vi "get_averaging_params_fd.vi"(7 "Current/sensor index":i32 min=0 max=1 step=1, 10 "Modulation info":T3 {"Hi channels at low" min=0 step=1; "Low carriers" format="%#_6p"; "High carriers" format="%#_6p"}, 11 "Config":T4={"IO params"={"Conversion"={"Rate"=4.0, "Num cards"=2, "Out channels"=4}, "Carriers"={"Phase shift"=180.0, "Levels"=[[0.8, 0.8, 0.8], [0.03, 0.03, 0.03]], "Delay samples"=73.15}, "TCP"={"Host"="192.168.1.15", "Port"=6666, "Buffering"=6, "Timeout"=6}, "Input channel sign"=[1, 1, 1]}, "High rate STFT"={"Win param"=101.5, "Window type"=61, "Win order"=2, "DFT size"=64, "Channels"=[7], "Oversample"=64}, "Low rate STFT"={"Win param"=120.0, "Window type"=61, "Win order"=8, "DFT size"=64, "Channels"=[7], "Oversample"=64}, "Filtering "=[]} {"Filtering"."Distortion"."Limit" format="%#_3p"; "Filtering"."Distortion"."LF cut" format="%#_3p"; "Filtering"."Kalman"."Measure noise" format="%#_3p"; "Filtering"."Kalman"."Process noise" format="%#_3p"; "Filtering"."Hum"."Limit" format="%#_3p"; "Filtering"."Hum"."Frequency" format="%#_4p"; "Low rate STFT"."Oversample" min=1 step=1; "Low rate STFT"."Channels" min=0 step=1; "Low rate STFT"."DFT size" min=1 step=1; "Low rate STFT"."Window type" items=["Rectangle"=0, "Hanning"=1, "Hamming"=2, "Blackman-Harris"=3, "Exact Blackman"=4, "Blackman"=5, "Flat Top"=6, "4 Term B-Harris "=7, "7 Term B-Harris"=8, "Low Sidelobe"=9, "Blackman Nuttall"=11, "Triangle"=30, "Bartlett-Hanning"=31, "Bohman"=32, "Parzen"=33, "Welch"=34, "Kaiser"=60, "Dolph-Chebyshev"=61, "Gaussian"=62]; "High rate STFT"."Oversample" min=1 step=1; "High rate STFT"."Channels" min=0 step=1; "High rate STFT"."DFT size" min=1 step=1; "High rate STFT"."Window type" items=["Rectangle"=0, "Hanning"=1, "Hamming"=2, "Blackman-Harris"=3, "Exact Blackman"=4, "Blackman"=5, "Flat Top"=6, "4 Term B-Harris "=7, "7 Term B-Harris"=8, "Low Sidelobe"=9, "Blackman Nuttall"=11, "Triangle"=30, "Bartlett-Hanning"=31, "Bohman"=32, "Parzen"=33, "Welch"=34, "Kaiser"=60, "Dolph-Chebyshev"=61, "Gaussian"=62]; "IO params"."Input channel sign" min=-1 max=1 step=1; "IO params"."Carriers"."Levels" min=0.0 step=0.1; "IO params"."Conversion"."Rate" format="%#_8g"}) -> (2 "Hum params":T1={"Order"=0, "Time constant"=0.0, "Detrend mode"=enum."Robust linear", "TD amplitude limit"=inf, "FFT filter"=TRUE, "Notch channels"=[], "LF cutoff"=0, "FD amplitude limit"=0.0}, 3 "Distortion params":T1={"Order"=0, "Time constant"=0.0, "Detrend mode"=enum."Robust linear", "TD amplitude limit"=inf, "FFT filter"=TRUE, "Notch channels"=[], "LF cutoff"=0, "FD amplitude limit"=0.0})   [LabVIEW 2026]
uses:
  averaging_filter_params.ctl
  detrend_mode.ctl
  ilemt_config.ctl
  system/IO_params.ctl
  stft_params.ctl
  <vilib>/Analysis/4window.llb/windowTd.ctl
  filter_params.ctl
  modulation_info.ctl
  <vilib>/Analysis/NI_AALPro.lvlib
panel:
  # "Index into Config.Filtering, 0=current sense, 1=sensor card"
  # "Get averaging filter parameters for the distortion and hum filters,\noperating at Fd demodulated output rate."
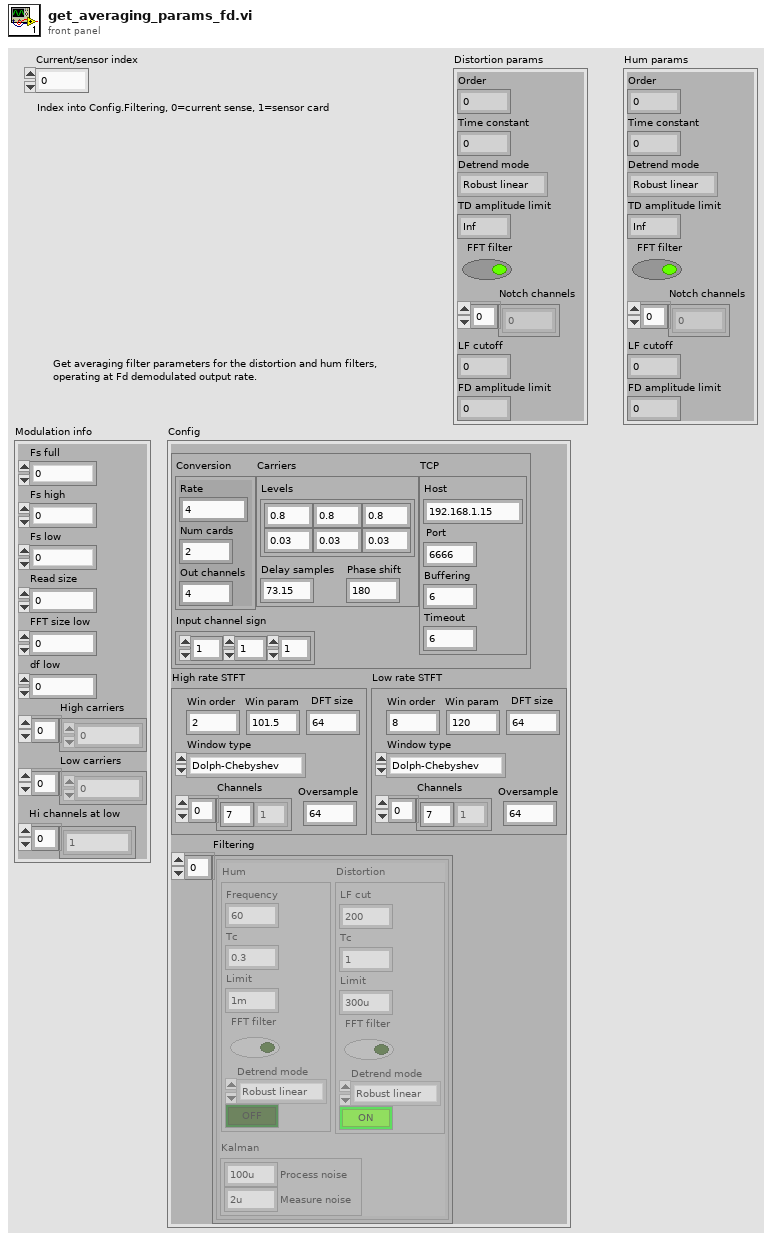
[diagram p1: front panel]
types:
  T1 = typedef "averaging_filter_params.ctl" = cluster{"Order":i32, "Time constant":dbl, "Detrend mode":T2, "TD amplitude limit":dbl, "FFT filter":bool, "Notch channels":i32[], "LF cutoff":i32, "FD amplitude limit":dbl}
  T2 = typedef "detrend_mode.ctl" = enum16{"Zero mean", "Linear", "Robust linear"}
  T3 = typedef "modulation_info.ctl" = cluster{"Fs full":dbl, "Fs high":dbl, "Fs low":dbl, "Read size":i32, "FFT size low":i32, "df low":dbl, "High carriers":dbl[], "Low carriers":dbl[], "Hi channels at low":i32[]}
  T4 = typedef "ilemt_config.ctl" = cluster{"IO params":T5, "High rate STFT":T6, "Low rate STFT":T6, "Filtering ":T8[]}
  T5 = typedef "IO_params.ctl" = cluster{"Conversion":cluster{"Rate":dbl, "Num cards":u32, "Out channels":u32}, "Carriers":cluster{"Phase shift":dbl, "Levels":dbl[][], "Delay samples":dbl}, "TCP":cluster{"Host":string, "Port":i32, "Buffering":u32, "Timeout":u32}, "Input channel sign":i32[]}
  T6 = typedef "stft_params.ctl" = cluster{"Win param":dbl, "Window type":T7, "Win order":i32, "DFT size":i32, "Channels":i32[], "Oversample":i32}
  T7 = typedef "NI_AALPro.lvlib/windowTd.ctl" = u32
  T8 = typedef "filter_params.ctl" = cluster{"Hum":cluster{"Frequency":dbl, "Tc":dbl, "Limit":dbl, "FFT filter":bool, "Detrend mode":T2, "Enable":bool}, "Kalman":cluster{"Process noise":dbl, "Measure noise":dbl}, "Distortion":cluster{"LF cut":dbl, "Tc":dbl, "Limit":dbl, "FFT filter":bool, "Detrend mode":T2, "Enable":bool}}
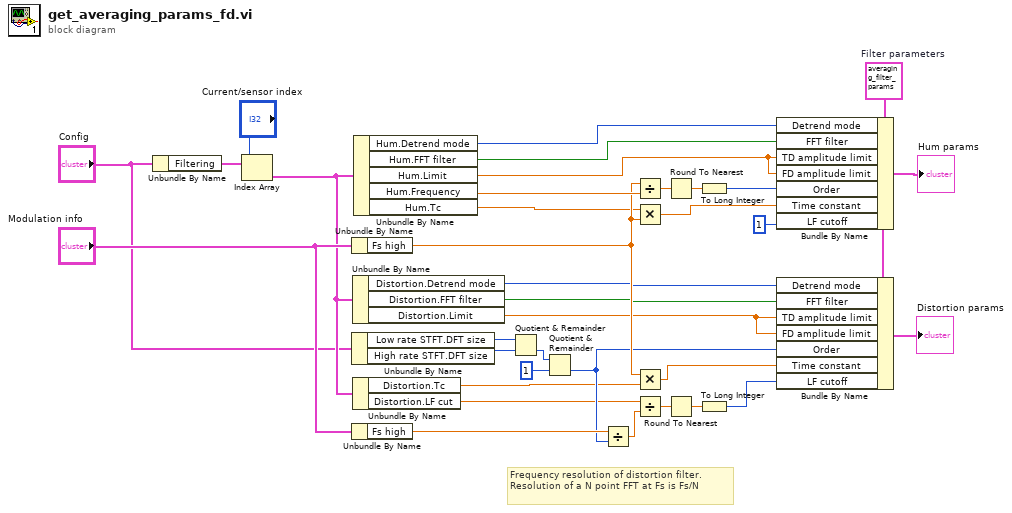
[diagram p0: block diagram]
diagram:
  w21 = T1 {"Order"=0, "Time constant"=0.0, "Detrend mode"=enum."Robust linear", "TD amplitude limit"=inf, "FFT filter"=TRUE, "Notch channels"=[], "LF cutoff"=0, "FD amplitude limit"=inf}  # Filter parameters
  # "Frequency resolution of distortion filter.   Resolution of a N point FFT at Fs is Fs/N"
  n1 = Unbundle By Name("Config") -> ("Filtering"=w11:T8[])
  n2 = Index Array(array=w11, index="Current/sensor index") -> (element=w9:T8)
  n3 = Unbundle By Name("Modulation info") -> ("Fs high"=w30:dbl)
  n4 = Unbundle By Name("Config") -> ("Low rate STFT.DFT size"=w5:i32, "High rate STFT.DFT size"=w4:i32)
  n5 = Unbundle By Name("Modulation info") -> ("Fs high"=w19:dbl)
  n6 = Unbundle By Name(w9) -> ("Distortion.Detrend mode"=w8:T2, "Distortion.FFT filter"=w7:bool, "Distortion.Limit"=w6:dbl)
  n7 = Unbundle By Name(w9) -> ("Distortion.Tc"=w3:dbl, "Distortion.LF cut"=w2:dbl)
  n8 = Unbundle By Name(w9) -> ("Hum.Detrend mode"=w15:T2, "Hum.FFT filter"=w16:bool, "Hum.Limit"=w17:dbl, "Hum.Frequency"=w33:dbl, "Hum.Tc"=w23:dbl)
  n9 = Quotient & Remainder(x=w5, y=w4) -> (floor(x/y)=w14:i32)  [unwired: 1 out]
  n10 = Quotient & Remainder(x=w14, y=1) -> (floor(x/y)=w13:i32)  [unwired: 1 out]
  n11 = Divide(x=w19, y=w13) -> (x/y=w18:dbl)
  n12 = Divide(x=w30, y=w33) -> (x/y=w22:dbl)
  n13 = Multiply(x=w23, y=w30) -> (x*y=w29:dbl)
  n14 = Multiply(x=w30, y=w3) -> (x*y=w28:dbl)
  n15 = Divide(x=w2, y=w18) -> (x/y=w34:dbl)
  n16 = Round To Nearest(number=w22) -> (nearest integer value=w24:dbl)
  n17 = Round To Nearest(number=w34) -> (nearest integer value=w35:dbl)
  n18 = To Long Integer(number=w24) -> (32bit integer=w25:i32)
  n19 = To Long Integer(number=w35) -> (32bit integer=w31:i32)
  n20 = Bundle By Name(cluster=w21, "Detrend mode"=w15, "FFT filter"=w16, "TD amplitude limit"=w17, "FD amplitude limit"=w17, "Order"=w25, "Time constant"=w29, "LF cutoff"=1) -> (→"Hum params":T1)
  n21 = Bundle By Name(cluster=w21, "Detrend mode"=w8, "FFT filter"=w7, "TD amplitude limit"=w6, "FD amplitude limit"=w6, "Order"=w13, "Time constant"=w28, "LF cutoff"=w31) -> (→"Distortion params":T1)
